vi "Selection Dialog.vi"(6 "Multi-Selection?":bool, 8 "error in (no error)":errorcluster, 9 "Initial Selection":string[](array[string]), 10 "Tree Items":string[](array[string]), 11 "Root Tag":string) -> (0 "error out":errorcluster, 1 "Canceled":bool, 3 "Selected Names":string[](array[string]))   [LabVIEW 2011, in "Engine Sim System Explorer.lvlib"]
doc: "Standard Channel Select Dialog that allows the user to select which TimeStamp channel to use for the header information."
uses:
  Engine Sim System Explorer.lvlib
panel:
  in  "Channels":string[](tree)
  in  "Cancel":bool
  in  "OK":bool
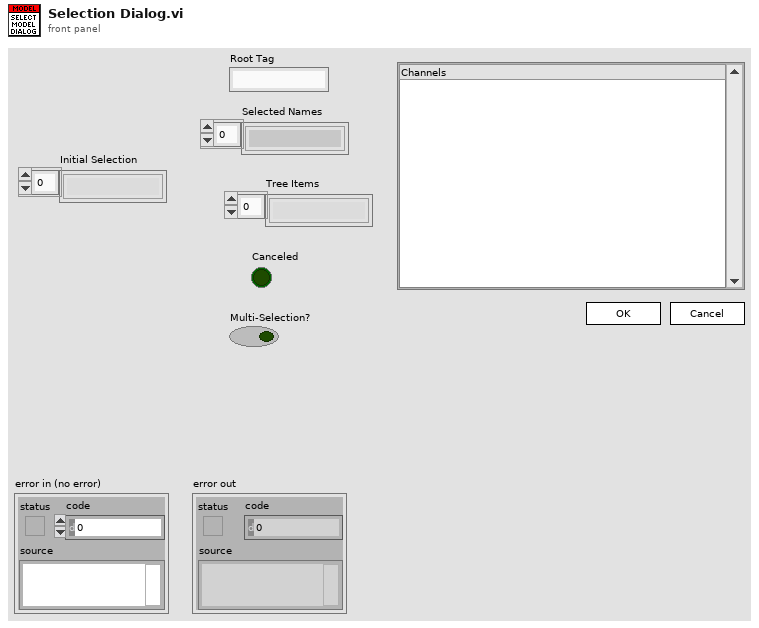
[diagram p1: front panel]
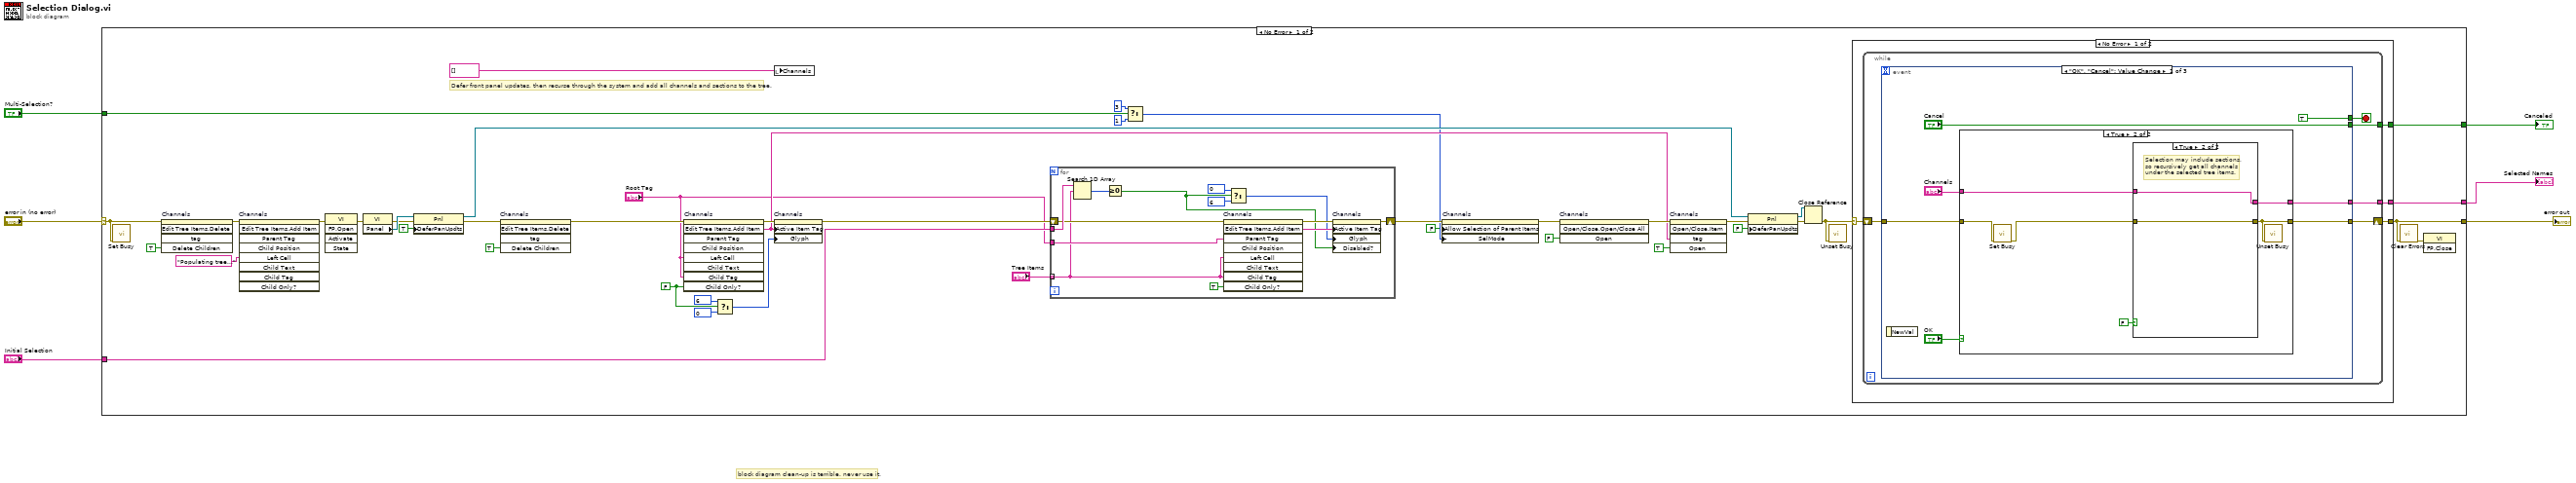
[diagram p0: block diagram]
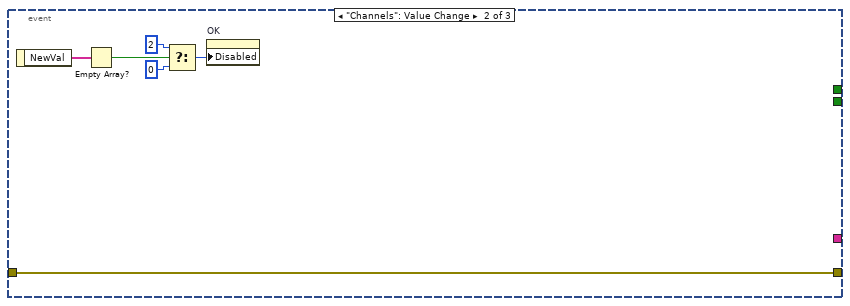
[diagram p4: hidden frame]
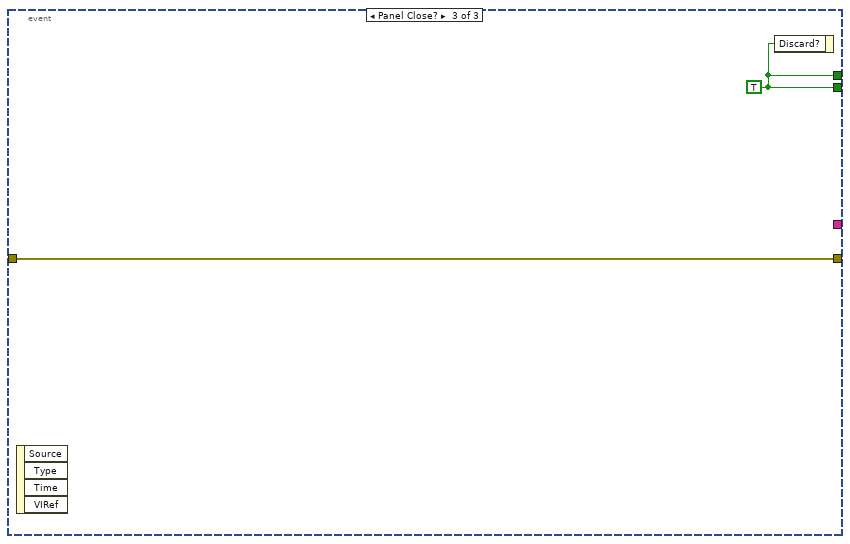
[diagram p5: hidden frame]
diagram:
  # "block diagram clean-up is terrible. never use it."
  n1 = case shown="No Error" "error in (no error)" {
    selector: "error in (no error)" -> [w18 w99]
    tunnel: "Initial Selection" -> [w19 _]
    tunnel: [w33 w99] -> w1
    tunnel: [w34 _] -> w4
    tunnel: [w31 _] -> w3
    tunnel: "Multi-Selection?" -> [w14 _]
    frame No Error {
      w10 = FALSE ("Is Channel")
      # "Defer front panel updates, then recurse through the system and add all channels and sections to the tree."
      n2 = call <vilib>:"Set Busy.vi"("error in (no error)"=w18) -> ()  [unwired: 3 in, 8 out]
      n3 = invoke on="Channels" class="Tree (strict)" method="Edit Tree Items.Delete"(error in=w18, "Delete Children"=TRUE ("Delete Children?")) -> (error out=w49:errorcluster)  [unwired: 3 in, 4 out]
      n4 = invoke on="Channels" class="Tree (strict)" method="Edit Tree Items.Add Item"(error in=w49, "Left Cell"="Populating tree..." ("Tag")) -> (error out=w46:errorcluster)  [unwired: 7 in, 8 out]
      n5 = invoke class="VI" method="FP.Open"(error in=w46) -> (error out=w44:errorcluster)  [unwired: 4 in, 4 out]
      n6 = property class="VI"(error in=w44) -> (error out=w42:errorcluster, "Panel"=w43:refnum<vi>)  [unwired: 1 in, 1 out]
      n7 = property class="Pnl"(reference=w43, error in=w42, "DeferPanUpdts"=TRUE ("Defer Panel Updates")) -> (reference out=w37:refnum<vi>, error out=w40:errorcluster)
      n8 = invoke on="Channels" class="Tree (strict)" method="Edit Tree Items.Delete"(error in=w40, "Delete Children"=TRUE ("Delete Children?")) -> (error out=w9:errorcluster)  [unwired: 3 in, 4 out]
      n9 = invoke on="Channels" class="Tree (strict)" method="Edit Tree Items.Add Item"(error in=w9, "Left Cell"="Root Tag", "Child Tag"="Root Tag", "Child Only?"=w10) -> (error out=w27:errorcluster, "Edit Tree Items:Add Item"=w22:string)  [unwired: 5 in, 7 out]
      n10 = Select(t=6, s=w10, f=0) -> (s? t:f=w30:i32)
      n11 = local write "Channels"(string[] [] ("Channels")) -> ()
      n12 = property on="Channels" class="Tree (strict)"(error in=w27, "Active Item Tag"=w22, "Glyph"=w30) -> (error out=w12:errorcluster)  [unwired: 1 in, 1 out]
      n13 = for {
        shift-right: [w59] -> w39
        shift-left: w12 -> [w52]
        tunnel: "Root Tag" -> [w62]
        tunnel: w19 -> [w55]
        tunnel: "Tree Items" -> [w51] mode=indexing
        n14 = Search 1D Array(1D array=w55, element=w51) -> (index of element=w54:i32)  [unwired: 1 in]
        n15 = Greater Or Equal To 0?(x=w54) -> (x >= 0?=w50:bool)
        n16 = invoke on="Channels" class="Tree (strict)" method="Edit Tree Items.Add Item"(error in=w52, "Parent Tag"=w62, "Left Cell"=w51, "Child Tag"=w51, "Child Only?"=TRUE) -> (error out=w61:errorcluster, "Edit Tree Items:Add Item"=w60:string)  [unwired: 4 in, 7 out]
        n17 = Select(t=0, s=w50, f=6) -> (s? t:f=w56:i32)
        n18 = property on="Channels" class="Tree (strict)"(error in=w61, "Active Item Tag"=w60, "Glyph"=w56, "Disabled?"=w50) -> (error out=w59:errorcluster)  [unwired: 1 in, 1 out]
      }
      n19 = Select(t=3 ("Selection Mode"), s=w14, f=1 ("Selection Mode")) -> (s? t:f=w15:i32)
      n20 = property on="Channels" class="Tree (strict)"(error in=w39, "Allow Selection of Parent Items"=FALSE, "SelMode"=w15) -> (error out=w26:errorcluster)  [unwired: 1 in, 1 out]
      n21 = invoke on="Channels" class="Tree (strict)" method="Open/Close.Open/Close All"(error in=w26, "Open"=FALSE ("Open?")) -> (error out=w24:errorcluster)  [unwired: 2 in, 3 out]
      n22 = invoke on="Channels" class="Tree (strict)" method="Open/Close.Item"(error in=w24, "tag"=w22, "Open"=TRUE ("Open?")) -> (error out=w20:errorcluster)  [unwired: 2 in, 4 out]
      n23 = property class="Pnl"(reference=w37, error in=w20, "DeferPanUpdts"=FALSE ("Defer Panel Updates")) -> (reference out=w35:refnum<vi>, error out=w36:errorcluster)
      n24 = Close Reference(reference=w35, error in (no error)=w36) -> (error out=w21:errorcluster)
      n25 = call <vilib>:"Unset Busy.vi"("error in (no error)"=w21) -> ()  [unwired: 1 in, 10 out]
      n26 = case shown="No Error" w21 {
        selector: w21 -> [w66 w98]
        tunnel: [w65 w98] -> w33
        tunnel: [w64 _] -> w34
        tunnel: [w63 _] -> w31
        frame No Error {
          n27 = while {
            shift-right: [w70] -> w65
            shift-left: w66 -> [w71]
            tunnel: [w69] -> w64
            tunnel: [w67] -> w63
            stop <- w68 stop-if-true
            n28 = event shown="[0] \"OK\", \"Cancel\": Value Change" {
              selector: _ -> [_ _ _]
              dyn-events: _ -> [_ _ _]
              timeout: _ -> [_ _ _]
              tunnel: w71 -> [w75 w95 w97]
              tunnel: [w73 w95 w97] -> w70
              tunnel: ["Cancel" _ w96] -> w69
              tunnel: [TRUE ("Discard?") _ w96] -> w68
              tunnel: [w74 _ _] -> w67
              event "OK", "Cancel": Value Change {
                n29 = event-data() -> ()  [unwired: 2 out]
                n30 = case shown="True" "OK" {
                  tunnel: "Channels" -> [_ w81]
                  tunnel: w75 -> [w79 w83]
                  tunnel: [_ w85] -> w74
                  tunnel: [w79 w84] -> w73
                  frame False {
                  }
                  frame True {
                    n31 = call <vilib>:"Set Busy.vi"("error in (no error)"=w83) -> ("error out"=w80:errorcluster)  [unwired: 3 in, 7 out]
                    n32 = case shown="True" FALSE {
                      tunnel: [w87 w89] -> w85
                      tunnel: [w86 w88] -> w84
                      tunnel: w81 -> [w87 w89]
                      tunnel: w80 -> [w86 w88]
                      frame False {
                      }
                      frame True {
                        # "Selection may include sections, so recursively get all channels under the selected tree items."
                      }
                    }
                    n33 = call <vilib>:"Unset Busy.vi"("error in (no error)"=w84) -> ()  [unwired: 1 in, 10 out]
                  }
                }
              }
              event "Channels": Value Change {
                n34 = event-data() -> ("NewVal"=w94:string[])  [unwired: 1 out]
                n35 = Empty Array?(array=w94) -> (empty?=w93:bool)
                n36 = Select(t=u8 2, s=w93, f=u8 0) -> (s? t:f=w90:u8)
                n37 = property on="OK" class="Bool"("Disabled"=w90) -> ()  [unwired: 2 in, 2 out]
              }
              event Panel Close? {
                w96 = TRUE ("Discard?")
                n38 = event-data() -> ()  [unwired: 5 out]
                n39 = event-data("Discard?"=w96) -> ()  [unwired: 1 in, 1 out]
              }
            }
          }
        }
        frame Error {
        }
      }
      n40 = call <vilib>:"Clear Errors.vi"("error in (no error)"=w33) -> ("error out"=w32:errorcluster)  [unwired: 6 out]
      n41 = invoke class="VI" method="FP.Close"(error in=w32) -> ()  [unwired: 2 in, 3 out]
    }
    frame Error {
    }
  }
  "Canceled" <- w4
  "Selected Names" <- w3
  "error out" <- w1
